vi "Settings Dialog.vi"(8 "error in (no error)":errorcluster caption="错误输入（无错误）", 11 "Configuration in":T1={"Hardware Configuration"={"Physical Channel"="", "Maximum Input"=0.0, "Minimum Input"=0.0, "Sample Rate"=0.0, "Number of Samples"=0}, "Analysis Configuration"={"Statistics"=TRUE}, "New Data Behavior"=enum."Replace"} caption="配置输入") -> (0 "error out":errorcluster caption="错误输出", 2 "UI Refresh Needed?":bool caption="需要刷新UI？", 3 "Configuration out":T1={"Hardware Configuration"={"Physical Channel"="", "Maximum Input"=0.0, "Minimum Input"=0.0, "Sample Rate"=0.0, "Number of Samples"=0}, "Analysis Configuration"={"Statistics"=TRUE}, "New Data Behavior"=enum."Replace"} caption="配置输出")   [LabVIEW 2013]
doc: "用于选择用户设置的对话框。"
uses:
  controls/User Specified Data.ctl
  controls/HW Configuration.ctl
  controls/Analysis Configuration.ctl
  controls/New Data Behavior.ctl
panel:
  in  "Number of Samples":i32=1000 caption="采样数"
  in  "Sample Rate":dbl=10000.0 caption="采样率"
  in  "Minimum Input":dbl=-10.0 caption="最小输入"
  in  "Maximum Input":dbl=10.0 caption="最大输入"
  in  "Physical Channel":tag="Dev1/ai0" caption="物理通道"
  in  "New Data Behavior":u16(ring) caption="新采集到数据时如何操作" items=["替换", "叠加", "添加"]
  in  "Cancel Button":bool caption="取消按钮"
  in  "OK Button":bool caption="确定按钮"
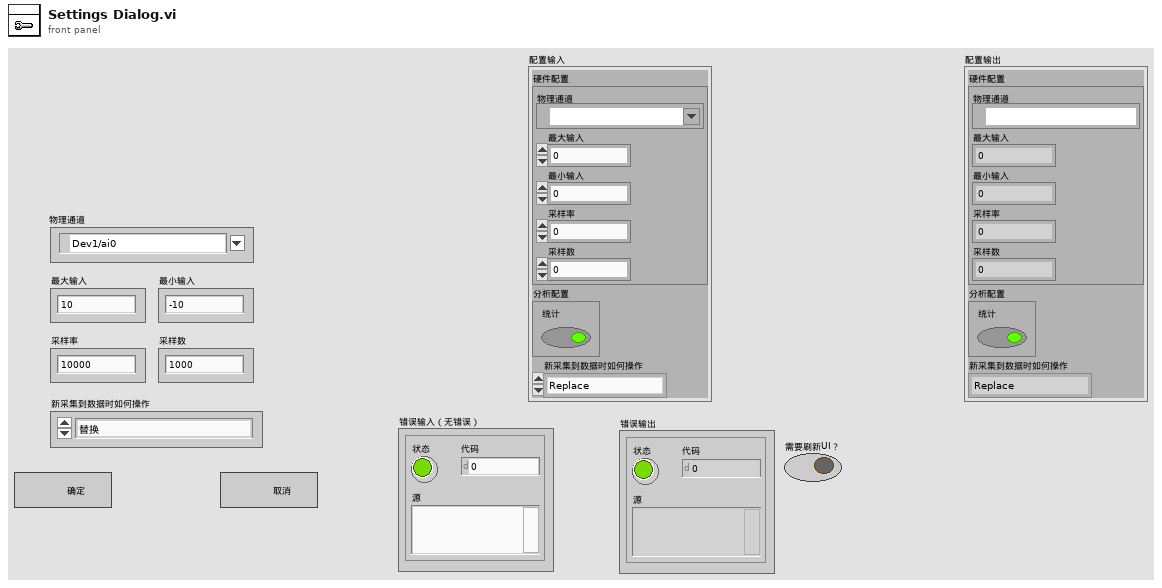
[diagram p1: front panel]
types:
  T1 = typedef "User Specified Data.ctl" = cluster{"Hardware Configuration":T2, "Analysis Configuration":T3, "New Data Behavior":T4}
  T2 = typedef "HW Configuration.ctl" = cluster{"Physical Channel":tag, "Maximum Input":dbl, "Minimum Input":dbl, "Sample Rate":dbl, "Number of Samples":i32}
  T3 = typedef "Analysis Configuration.ctl" = cluster{"Statistics":bool}
  T4 = typedef "New Data Behavior.ctl" = enum16{"Replace", "Overlay", "Append"}
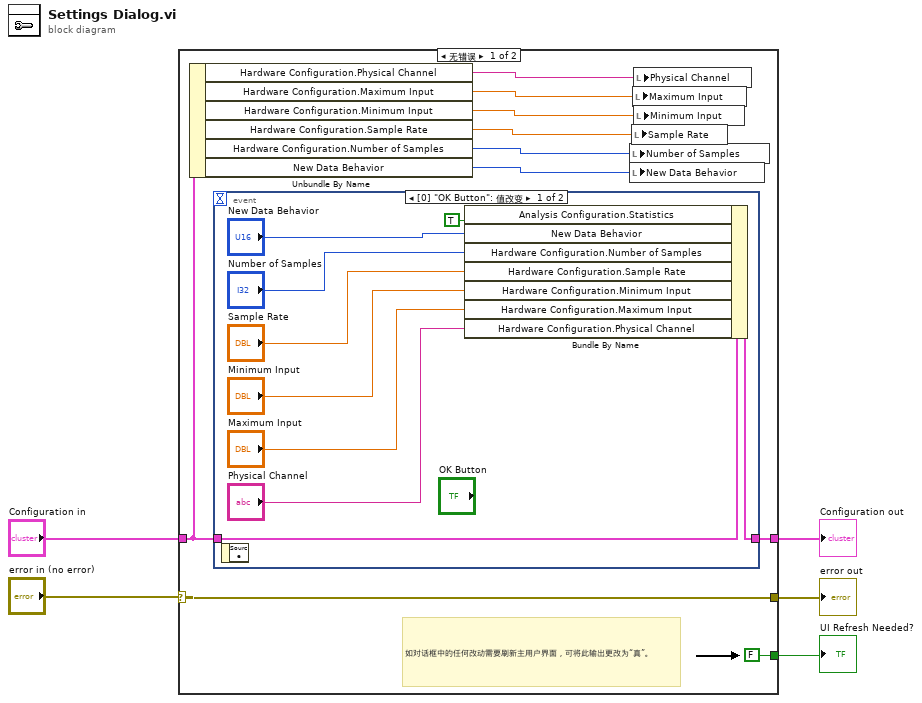
[diagram p0: block diagram]
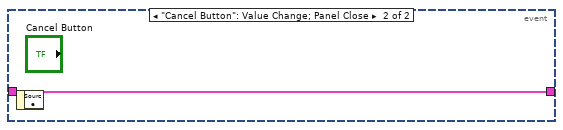
[diagram p2: hidden frame]
diagram:
  n1 = case shown="无错误" "error in (no error)" {
    selector: "error in (no error)" -> [w13 w27]
    tunnel: [w13 w27] -> w4
    tunnel: "Configuration in" -> [w12 w26]
    tunnel: [w15 w26] -> w2
    tunnel: [FALSE ("UI Refresh Needed?") _] -> w1
    frame No Error {
      # "如对话框中的任何改动需要刷新主用户界面，可将此输出更改为“真”。"
      n2 = Unbundle By Name(w12) -> ("Hardware Configuration.Physical Channel"=w11:tag, "Hardware Configuration.Maximum Input"=w10:dbl, "Hardware Configuration.Minimum Input"=w9:dbl, "Hardware Configuration.Sample Rate"=w8:dbl, "Hardware Configuration.Number of Samples"=w7:i32, "New Data Behavior"=w6:T4)
      n3 = event shown="[0] \"OK Button\": 值改变" {
        selector: _ -> [_ _]
        dyn-events: _ -> [_ _]
        timeout: _ -> [_ _]
        tunnel: [w24 w25] -> w15
        tunnel: w12 -> [w22 w25]
        event "OK Button": Value Change {
          n4 = event-data() -> ()  [unwired: 1 in, 1 out]
          n5 = Bundle By Name(cluster=w22, "Analysis Configuration.Statistics"=TRUE, "New Data Behavior"="New Data Behavior", "Hardware Configuration.Number of Samples"="Number of Samples", "Hardware Configuration.Sample Rate"="Sample Rate", "Hardware Configuration.Minimum Input"="Minimum Input", "Hardware Configuration.Maximum Input"="Maximum Input", "Hardware Configuration.Physical Channel"="Physical Channel") -> (w24:T1)
        }
        event "Cancel Button": Value Change; Panel Close {
          n6 = event-data() -> ()  [unwired: 1 in, 1 out]
        }
      }
      n7 = local write "Number of Samples"(w7) -> ()
      n8 = local write "New Data Behavior"(w6) -> ()
      n9 = local write "Sample Rate"(w8) -> ()
      n10 = local write "Maximum Input"(w10) -> ()
      n11 = local write "Physical Channel"(w11) -> ()
      n12 = local write "Minimum Input"(w9) -> ()
    }
    frame Error {
    }
  }
  "UI Refresh Needed?" <- w1
  "error out" <- w4
  "Configuration out" <- w2
